vi "Auto Jump.vi"(11 "Condition":dbl) -> (3 "Jump?":bool)   [LabVIEW 2015]
uses:
  Robot Global Data.vi
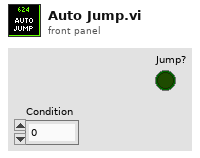
[diagram p1: front panel]
types:
  T1 = typedef "Dashboard Control Data.ctl" = cluster{"Shooter Presets":T2, "Encoder Control":T4, "Steer PID output":cluster{"output high":dbl, "output low":dbl}, " Steer PID gains":cluster{"proportional gain (Kc)":dbl, "integral time (Ti, min)":dbl, "derivative time (Td, min)":dbl}, "Drivetrain Settings":T5, "Vision Packet":T6, "Dashboard Drivetrain Command":T7, "Info/Command Cluster":T9, "Ball Vision Packet":T10, "Intake Presets":T12, "Intake Encoder Control":T14, "Climb Presets":T15, "Goal Output Range":cluster{"output high":dbl, "output low":dbl}, "Enabled Systems":T16, "Auton Presets":T17}
  T2 = typedef "Shooter Presets.ctl" = cluster{"Batter Shot":T3, "Deep Middle Shot":T3, "Manual Shot":T3, "Left Ticks Per Rotation":dbl, "Right Ticks Per Rotation":dbl, "Low Bar Shot":T3, "Shooter RPM Tolerance":dbl, "IIR Filter Power":dbl, "Trigger Power":dbl, "Fire from Load Delay":i32, "Max Angle":dbl, "Min Angle":dbl, "Angle PID gains":cluster{"P":dbl, "I":dbl, "D":dbl}, "Angle Output":cluster{"output high":dbl, "output low":dbl}, "Shooter Angle Tolerance":dbl, "Vision Shoot x^2":dbl, "Vision Shoot x":dbl, "Dist from Axis Cam to Pivot":dbl, "High Goal Center Height":dbl, "Feed Forward Max Accel":dbl, "Feed Forward Kv":dbl, "Backwards Trigger":dbl, "Shot Finish Delay (ms)":dbl, "Angle Max Current":dbl, "Angle Current Trip Time":dbl, "Intake Angle":dbl, "Vision Shoot c":dbl, "Reset?":bool, "Servo Release Delay":dbl, "Servo Idle Angle":i32, "Servo Hold Angle":i32, "Angle Pot x":dbl, "Angle Pot c":dbl, "Ignore Angle?":bool, "Manual Output?":bool, "Manual Out":dbl, "Max RPM":dbl, "Safty Frist Angle":dbl, "Intake Danger Height":dbl, "Angle Pot B":i32, "Angle Pot M":dbl, "FF Finish RPM":dbl, "RPM PID Right":cluster{"P":dbl, "I":dbl, "D":dbl, "FF":dbl}, "RPM PID Left":cluster{"P":dbl, "I":dbl, "D":dbl, "FF":dbl}, "Backwards RPM":dbl}
  T3 = typedef "Shot Presets.ctl" = cluster{"Left":dbl, "Right":dbl, "Angle":dbl}
  T4 = typedef "Encoder Control.ctl" = cluster{"Right Tick Constant":dbl, "Left Tick Constant":dbl, "Reset?":bool, "Y Dist":cluster{"PID gains":cluster{"proportional gain (Kc)":dbl, "integral time (Ti, min)":dbl, "derivative time (Td, min)":dbl}}, "Y Stop Thresh":dbl, "Y Stop Speed":dbl}
  T5 = typedef "Drivetrain Settings.ctl" = cluster{"Gyro Tolerance":dbl, "Throttle Ramp (ms)":dbl, "Angular rate compensation":bool, "Throttle to Rate Scale":dbl, "Rate compensation gain":dbl, "Kv":dbl, "Ka":dbl, "Feed Forward P":dbl, "Feed Forward D":dbl, "Goal Vision PID gains":cluster{"proportional gain (Kc)":dbl, "integral time (Ti, min)":dbl, "derivative time (Td, min)":dbl}, "Goal Detection Window":dbl, "Creep Rate":dbl}
  T6 = typedef "Goal Vision Packet.ctl" = cluster{"Distance":dbl, "Center X":dbl, "Center Y":dbl, "Found Target?":bool}
  T7 = typedef "Dashboard Drivetrain Command.ctl" = cluster{"Drivetrain Vision":T8}
  T8 = typedef "Drivetrain Vision.ctl" = cluster{"Goal Window":dbl, "Ball Window":dbl}
  T9 = typedef "Ball Tracking Command Cluster.ctl" = cluster{"Distance to Ball":dbl, "Desired Angle":dbl, "Command":enum16{"Turn to Ball", "Turn to Angle", "Get Distance"}, "Pixels from Center":dbl}
  T10 = typedef "Ball Vision Packet.ctl" = cluster{"Ball Detected?":bool, "Distance to Ball":dbl, "Desired Angle":dbl, "Pixels from Center":dbl, "Tracking mode":T11}
  T11 = typedef "Tracking Mode.ctl" = enum16{"Turn to Ball", "Turn to Angle"}
  T12 = typedef "Intake Presets.ctl" = cluster{"Intake Speed":dbl, "Outake Speed":dbl, "Low Height":dbl, "Half Height":dbl, "Full Height":dbl, "Angle Speed":dbl, "Angle Tolerance":dbl, "Encoder Scale":dbl, "Load Height":dbl, "Output Range":T13, "Rotation Power Max/Min":dbl, "MaxCurrent":dbl, "Intake Trip Time":dbl, "Idle Height":dbl, "Max Height":dbl, "Reset Encoders?":bool, "PID gains":cluster{"proportional gain (Kc)":dbl, "integral time (Ti, min)":dbl, "derivative time (Td, min)":dbl}}
  T13 = typedef "Drivetrain Output Range.ctl" = cluster{"output high":dbl, "output low":dbl}
  T14 = typedef "IntakeEcoderControl.ctl" = cluster{"Arm Tick Constant":dbl, "Reset?":bool, "Y Dist":cluster{"PID gains":cluster{"proportional gain (Kc)":dbl, "integral time (Ti, min)":dbl, "derivative time (Td, min)":dbl}}, "Y Stop Thresh":dbl, "Y Stop Speed":dbl}
  T15 = typedef "Climb Presets.ctl" = cluster{"Pull Power":dbl, "Unpin Power":dbl, "Time to Hold":dbl, "Extend Power":dbl}
  T16 = typedef "Enabled Systems.ctl" = cluster{"Shoot":bool, "Intake":bool, "DT":bool, "Gyro":bool, "100ms":bool, "US":bool}
  T17 = typedef "Autonomous Presets.ctl" = cluster{"Pitch Limit":dbl, "Roll Limit":dbl, "Ultrasonic Limit":dbl, "Start Position":dbl, "Cross Position":dbl}
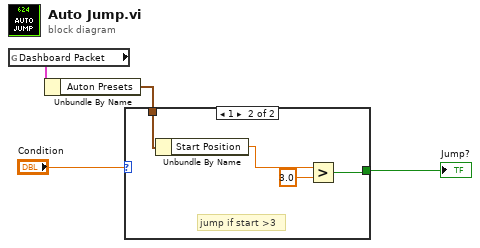
[diagram p0: block diagram]
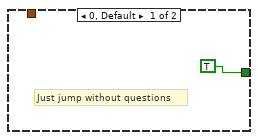
[diagram p2: hidden frame]
diagram:
  n1 = global read "Robot Global Data.vi" "Dashboard Packet"() -> (w2:T1)
  n2 = Unbundle By Name(w2) -> ("Auton Presets"=w1:T17)
  n3 = case shown="1" "Condition" {
    tunnel: [TRUE w6] -> w3
    tunnel: w1 -> [_ w9]
    frame 0, Default {
      # "Just jump without questions"
    }
    frame 1 {
      # "jump if start >3"
      n4 = Unbundle By Name(w9) -> ("Start Position"=w8:dbl)
      n5 = Greater?(x=w8, y=3.0) -> (0:w6:bool)
    }
  }
  "Jump?" <- w3
